vi "I32 to U64.vi"(1 "I32":i32) -> (0 "U64 cast as DBL":dbl)   [LabVIEW 2017]
panel:
  # "LVHDF5 Toolkit\nCopyright (c) 2005-2013 by Jason D. Sommerville\nCopyright (c) 2014 by UPVI, LLC.\n\nThis use and distribution of this file is governed by the terms found in \nLICENSE.txt distributed with this toolkit and installed at\n <user.lib>\\_lvhdf5\\LICENSE.txt"
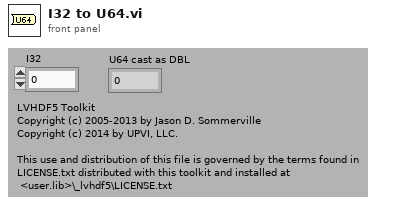
[diagram p1: front panel]
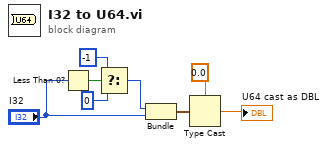
[diagram p0: block diagram]
diagram:
  n1 = Less Than 0?(x="I32") -> (x < 0?=w8:bool)
  n2 = Select(t=-1, s=w8, f=0) -> (s? t:f=w4:i32)
  n3 = Bundle(w4, "I32"="I32") -> (w3:cluster{i32, "I32":i32})  [unwired: 1 in]
  n4 = Type Cast(type=0.0, x=w3) -> (*(type *) &x=→"U64 cast as DBL":dbl)
